vi "GetPictureData(16).vi"(5 "Resolution":cluster{"Width":u32, "Height":u32}, 6 "Data(16Bit)":u16[](array[numeric]), 7 "ColorType":enum16{"MONO", "COLOR"}(ring)) -> (3 "new picture":picture)   [LabVIEW 2015]
uses:
  <vilib>/picture/picture.llb/imagedata.ctl
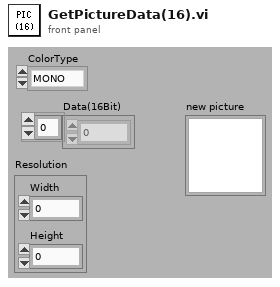
[diagram p1: front panel]
types:
  T1 = typedef "imagedata.ctl" = cluster{"image type":i32, "image depth":i32, "image":u8[], "mask":u8[], "colors":u32[], "Rectangle":cluster{"left":i16, "top":i16, "right":i16, "bottom":i16}}
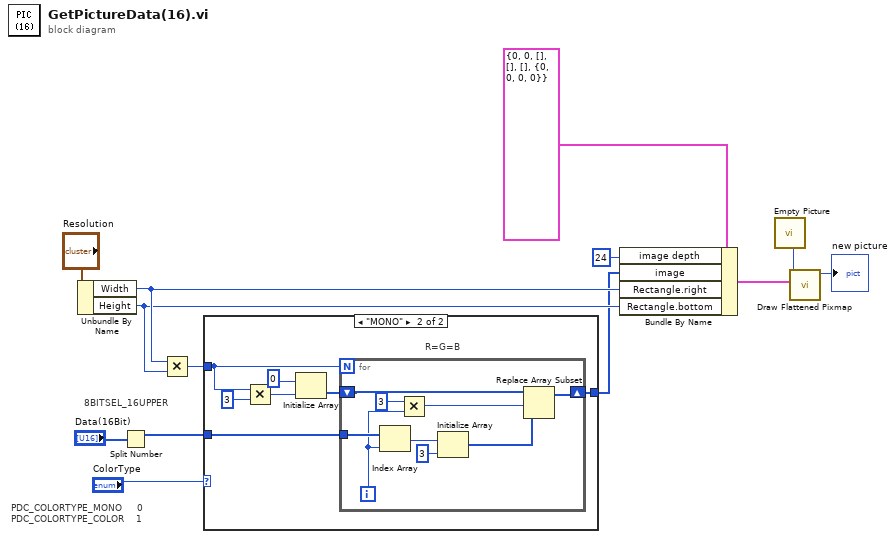
[diagram p0: block diagram]
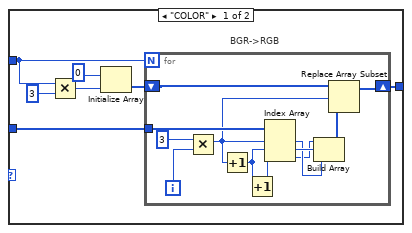
[diagram p2: hidden frame]
diagram:
  # "8BITSEL_16UPPER"
  # "PDC_COLORTYPE_MONO\t\t\t\t\t0\nPDC_COLORTYPE_COLOR\t\t\t\t1"
  n1 = Unbundle By Name("Resolution") -> ("Width"=w9:u32, "Height"=w8:u32)
  n2 = Split Number(x="Data(16Bit)") -> (hi(x)=w1:u8[])  [unwired: 1 out]
  n3 = Multiply(x=w9, y=w8) -> (x*y=w10:u32)
  n4 = case shown="\"MONO\"" "ColorType" {
    tunnel: w10 -> [w19 w38]
    tunnel: [w15 w34] -> w7
    tunnel: w1 -> [w14 w33]
    frame "COLOR" {
      # "BGR->RGB"
      n5 = Multiply(x=w19, y=3) -> (x*y=w17:u32)
      n6 = Initialize Array(u16 0, w17) -> (w16:u16[])
      n7 = for {
        N: w19 -> [_]
        shift-right: [w23] -> w15
        shift-left: w16 -> [w24]
        tunnel: w14 -> [w32]
        i -> [w27]
        n8 = Multiply(x=3, y=w27) -> (x*y=w21:i32)
        n9 = Increment(x=w21) -> (x+1=w26:i32)
        n10 = Increment(x=w26) -> (x+1=w25:i32)
        n11 = Index Array(array=w32, index #1=w21, index #2=w26, index #3=w25) -> (element #1=w30:u8, element #2=w31:u8, element #3=w29:u8)
        n12 = Build Array(w29, w31, w30) -> (w22:u8[])
        n13 = Replace Array Subset(array=w24, new element=w22, index=w21) -> (w23:u16[])
      }
    }
    frame "MONO" {
      # "R=G=B"
      n14 = Multiply(x=w38, y=3) -> (x*y=w36:u32)
      n15 = Initialize Array(u16 0, w36) -> (w35:u16[])
      n16 = for {
        N: w38 -> [_]
        shift-right: [w45] -> w34
        shift-left: w35 -> [w46]
        tunnel: w33 -> [w48]
        i -> [w43]
        n17 = Index Array(array=w48, index=w43) -> (element=w42:u8)
        n18 = Multiply(x=3, y=w43) -> (x*y=w44:i32)
        n19 = Initialize Array(w42, 3 ("次元サイズ")) -> (w40:u8[])
        n20 = Replace Array Subset(array=w46, new element=w40, index=w44) -> (w45:u16[])
      }
    }
  }
  n21 = Bundle By Name(cluster=T1 {"image type"=0, "image depth"=0, "image"=[], "mask"=[], "colors"=[], "Rectangle"={"left"=0, "top"=0, "right"=0, "bottom"=0}} ("image data"), "image depth"=24, "image"=w7, "Rectangle.right"=w9, "Rectangle.bottom"=w8) -> (w13:T1)
  n22 = call "Empty Picture"() -> ("empty picture"=w3:picture)
  n23 = call <vilib>:"Draw Flattened Pixmap.vi"("image data"=w13, "picture"=w3) -> ("new picture"=→"new picture":picture)  [unwired: 7 out]
